vi "EnqueueResponse.vi"(0 "cmdRef in":T1, 5 "response":string, 11 "error in (no error)":errorcluster) -> (4 "cmdRef out":T1, 15 "error out":errorcluster)   [LabVIEW 2017, in "vsws.lvlib"]
uses:
  vsws.lvlib
  cmdRef.ctl
  cmd.ctl
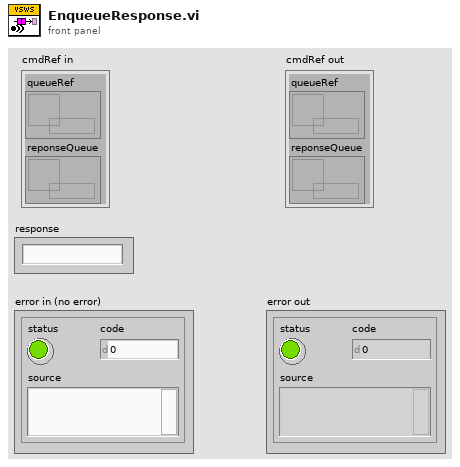
[diagram p1: front panel]
types:
  T1 = typedef "vsws.lvlib/cmdRef.ctl" = cluster{"queueRef":refnum<queue>, "reponseQueue":refnum<queue>}
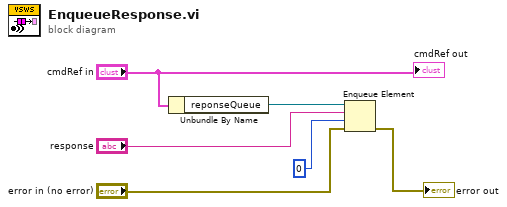
[diagram p0: block diagram]
diagram:
  n1 = Unbundle By Name("cmdRef in") -> ("reponseQueue"=w5:refnum<queue>)
  n2 = Enqueue Element(queue=w5, element="response", timeout in ms (-1)=0, error in (no error)="error in (no error)") -> (error out=→"error out":errorcluster)  [unwired: 2 out]
  "cmdRef out" <- "cmdRef in"
